vi "Untitled 2.vi"() -> ()   [LabVIEW 2015]
panel:
  in  "Shared Variable Control":refnum<k21>
  out "error out":errorcluster
  out "data":dbl
  out "Baratron 1":dbl(knob) scale=0.0005..1000.0
  in  "Vertical Pointer Slide 2":dbl(slide) scale=-1.0..1.0
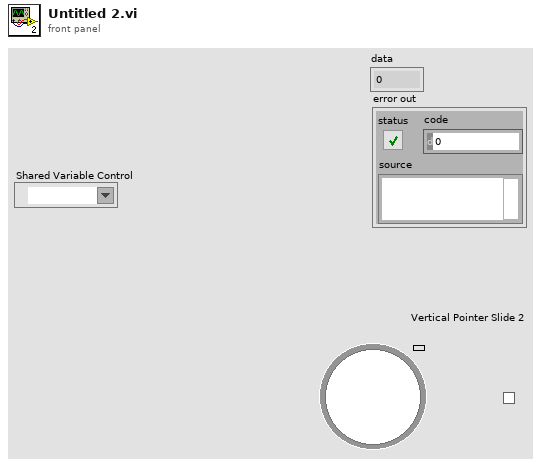
[diagram p1: front panel]
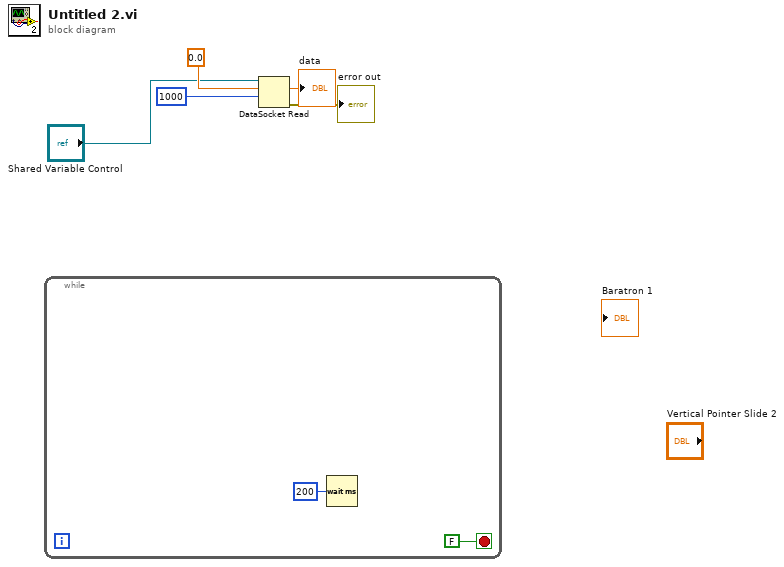
[diagram p0: block diagram]
diagram:
  n1 = while {
    stop <- FALSE stop-if-true
    n2 = Wait (ms)(milliseconds to wait=u32 200) -> ()  [unwired: 1 out]
  }
  n3 = DataSocket Read(9:1000 ("ms timeout (10000)"), 10:0.0, 11:"Shared Variable Control") -> (0:→"error out":errorcluster, 2:→"data":dbl)  [unwired: 2 in, 5 out]
